vi "mW_CheckFreq.vi"(9 "Range(GHz)":dbl, 10 "Center Frequency(GHz)":dbl=140.18, 11 "Current Frequency":dbl) -> (0 "Lower":dbl, 2 "Freq_in Range":bool, 3 "Upper":dbl)   [LabVIEW 2019]
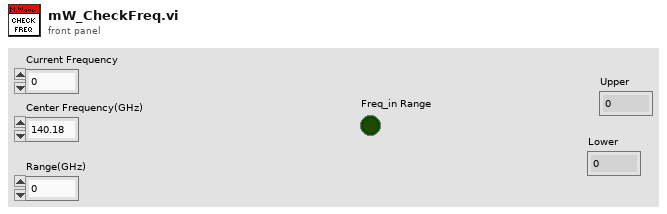
[diagram p1: front panel]
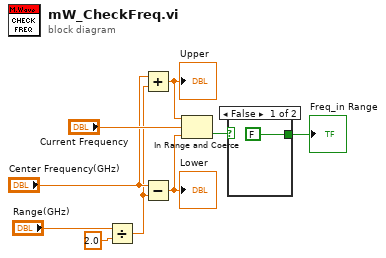
[diagram p0: block diagram]
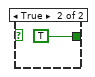
[diagram p2: hidden frame]
diagram:
  n1 = Divide(x="Range(GHz)", y=2.0) -> (x/y=w4:dbl)
  n2 = Add(x="Center Frequency(GHz)", y=w4) -> (x+y=w6:dbl)
  "Upper" <- w6
  n3 = Subtract(x="Center Frequency(GHz)", y=w4) -> (x-y=w3:dbl)
  "Lower" <- w3
  n4 = In Range and Coerce(upper limit=w6, x="Current Frequency", lower limit=w3) -> (In Range?=w2:bool)  [unwired: 1 out]
  n5 = case shown="False" w2 {
    tunnel: [FALSE ("Freq_in Range") TRUE ("Freq_in Range")] -> w1
    frame False {
    }
    frame True {
    }
  }
  "Freq_in Range" <- w1
